vi "Semaphore Kaushik.vi"() -> ()   [LabVIEW 2022 SP3]
panel:
  out "DATA 2 LOOP 2":dbl(graph)
  out "DATA 1 LOOP 1":dbl(graph)
  out "Loop 2 Access":bool
  out "Loop 1 Access":bool
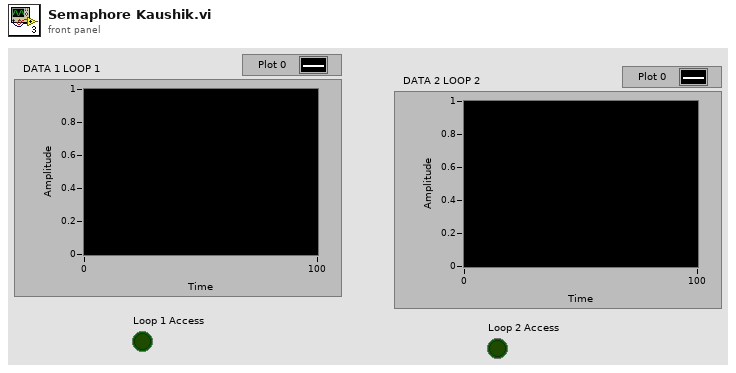
[diagram p1: front panel]
types:
  T1 = typedef "Semaphore RefNum" = refnum<k1>
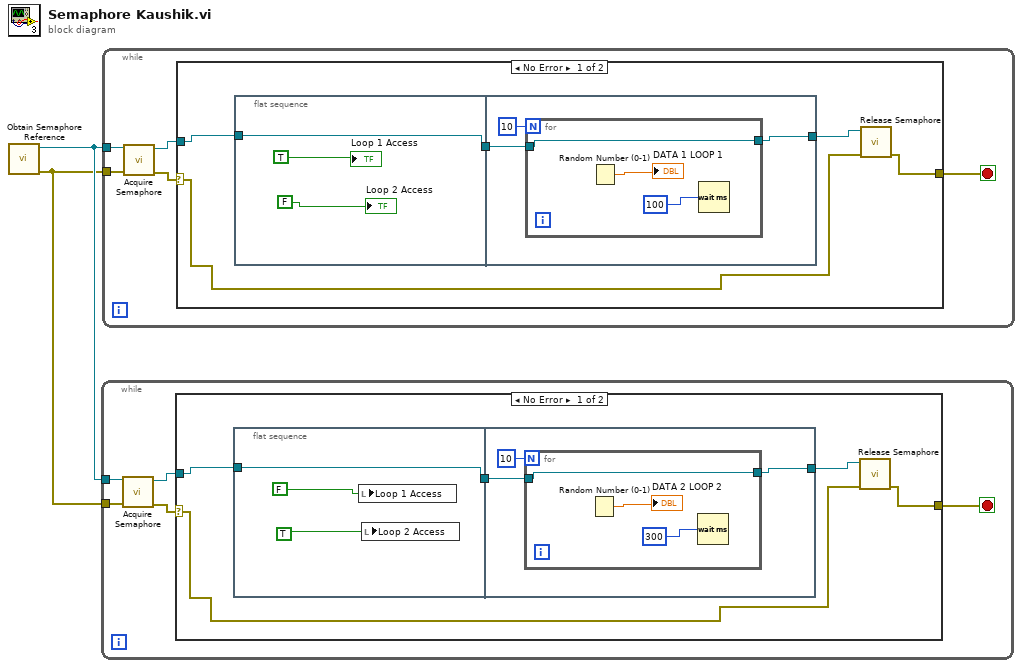
[diagram p0: block diagram]
diagram:
  n1 = call <vilib>:"Obtain Semaphore Reference.vi"() -> ("error out"=w1:errorcluster, "semaphore"=w2:T1)  [unwired: 5 in, 1 out]
  n2 = while {
    tunnel: w1 -> [w7]
    tunnel: w2 -> [w6]
    stop <- w3 stop-if-true
    n3 = call <vilib>:"Acquire Semaphore.vi"("error in (no error)"=w7, "semaphore"=w6) -> ("error out"=w4:errorcluster, "semaphore out"=w5:T1)  [unwired: 3 in, 1 out]
    n4 = case shown="No Error" w4 {
      selector: w4 -> [w9 w22]
      tunnel: w5 -> [w12 _]
      tunnel: [w8 w22] -> w3
      frame No Error {
        n5 = flat-sequence {
          tunnel: w12 -> [w15]
          tunnel: [w15] -> w11
          tunnel: w11 -> [w17]
          tunnel: [w16] -> w10
          frame #0 {
            n6 = local write "Loop 1 Access"(FALSE) -> ()
            n7 = local write "Loop 2 Access"(TRUE) -> ()
          }
          frame #1 {
            n8 = for {
              N: 10 -> [_]
              tunnel: [w19] -> w16
              tunnel: w17 -> [w19]
              n9 = Random Number (0-1)() -> (number: 0 to 1=→"DATA 2 LOOP 2":dbl)
              n10 = Wait (ms)(milliseconds to wait=u32 300) -> ()  [unwired: 1 out]
            }
          }
        }
        n11 = call <vilib>:"Release Semaphore.vi"("error in (no error)"=w9, "semaphore"=w10) -> ("error out"=w8:errorcluster)  [unwired: 4 in, 1 out]
      }
      frame Error {
      }
    }
  }
  n12 = while {
    tunnel: w1 -> [w27]
    tunnel: w2 -> [w26]
    stop <- w23 stop-if-true
    n13 = call <vilib>:"Acquire Semaphore.vi"("error in (no error)"=w27, "semaphore"=w26) -> ("error out"=w24:errorcluster, "semaphore out"=w25:T1)  [unwired: 3 in, 1 out]
    n14 = case shown="No Error" w24 {
      selector: w24 -> [w29 w42]
      tunnel: w25 -> [w32 _]
      tunnel: [w28 w42] -> w23
      frame No Error {
        n15 = flat-sequence {
          tunnel: w32 -> [w33]
          tunnel: [w33] -> w31
          tunnel: w31 -> [w37]
          tunnel: [w36] -> w30
          frame #0 {
            "Loop 1 Access" <- TRUE
            "Loop 2 Access" <- FALSE
          }
          frame #1 {
            n16 = for {
              N: 10 -> [_]
              tunnel: [w39] -> w36
              tunnel: w37 -> [w39]
              n17 = Random Number (0-1)() -> (number: 0 to 1=→"DATA 1 LOOP 1":dbl)
              n18 = Wait (ms)(milliseconds to wait=u32 100) -> ()  [unwired: 1 out]
            }
          }
        }
        n19 = call <vilib>:"Release Semaphore.vi"("error in (no error)"=w29, "semaphore"=w30) -> ("error out"=w28:errorcluster)  [unwired: 4 in, 1 out]
      }
      frame Error {
      }
    }
  }
